vi "ifr2025 Phase.vi"(8 "error in (no error)":errorcluster {"code" format="%.0x"}, 9 "Carrier Phase (0.0)":dbl, 11 "instrument handle":refnum<visa-resource-name>) -> (0 "error out":errorcluster {"code" format="%.0x"}, 3 "instrument handle out":refnum<visa-resource-name>)   [LabVIEW 2009]
doc: "Adjust the phase offset of the carrier."
uses:
  Ifr2025_32.dll
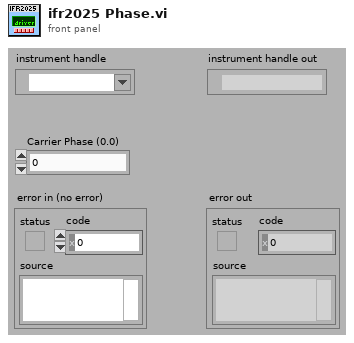
[diagram p1: front panel]
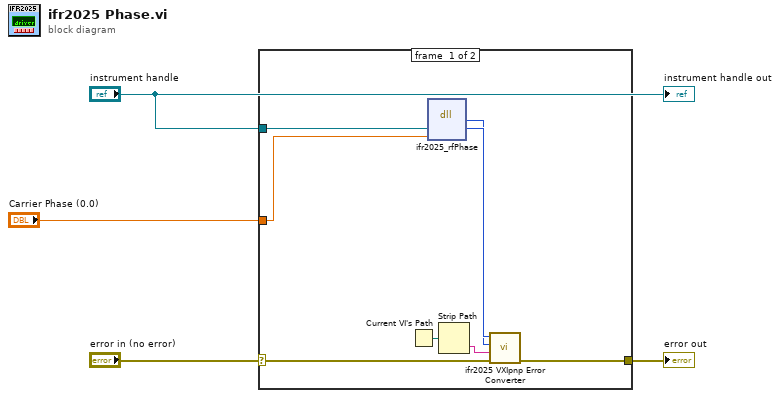
[diagram p0: block diagram]
diagram:
  n1 = case shown="No Error" "error in (no error)" {
    selector: "error in (no error)" -> [w7 w13]
    tunnel: [w6 w13] -> w4
    tunnel: "instrument handle" -> [w11 _]
    tunnel: "Carrier Phase (0.0)" -> [w5 _]
    frame #0 {
      n2 = Current VI's Path() -> (path=w12:path)
      n3 = dll-call lib="P:/inst/Marconi 2024 Signal Generator/source/labview/ifr2025/ifr2025/ifr2025_*.*" fn="ifr2025_rfPhase"("vi"=w11, "Carrier Phase"=w5) -> (w9:i32, "vi"=w10:u32)  [unwired: 4 in, 2 out]
      n4 = Strip Path(path=w12) -> (name=w8:string)  [unwired: 1 out]
      n5 = call "ifr2025 VXIpnp Error Converter.vi"("error in (no error)"=w7, "name of VI (\"\")"=w8, "CVI error code (0)"=w9, "instrument handle"=w10) -> ("error out"=w6:errorcluster)  [unwired: 7 out]
    }
    frame #1 {
    }
  }
  "error out" <- w4
  "instrument handle out" <- "instrument handle"
